vi "Actor Core.vi"(8 "error in":errorcluster, 11 "SCHEMA_01 in":refnum<class "SCHEMA_01.lvclass">) -> (0 "error out":errorcluster, 3 "Actor out":refnum<class "Actor.lvclass">)   [LabVIEW 2020, in "SCHEMA_01.lvlib" / "SCHEMA_01.lvclass"]
uses:
  SCHEMA_01.lvclass
  support/Actor Framework.lvlibp/1abvi3w/vi.lib/ActorFramework/Actor/Actor.lvclass
  D&C_SchemaBase/D&C_SchemaBase/D&C_SchemaBase.lvclass
panel:
  out "Source 1.T_0":dbl caption="Random.VAR 1" format="%#.1f"
  out "Source 1.T_6":dbl caption="Random.VAR 1" format="%#.1f"
  out "Source 1.T_5":dbl caption="Random.VAR 1" format="%#.1f"
  out "Source 1.T_4":dbl caption="Random.VAR 1" format="%#.1f"
  out "Source 1.T_3":dbl caption="Random.VAR 1" format="%#.1f"
  out "Source 1.T_2":dbl caption="Random.VAR 1" format="%#.1f"
  out "Source 1.T_1":dbl caption="Random.VAR 1" format="%#.1f"
  # "Source 1: les températures"
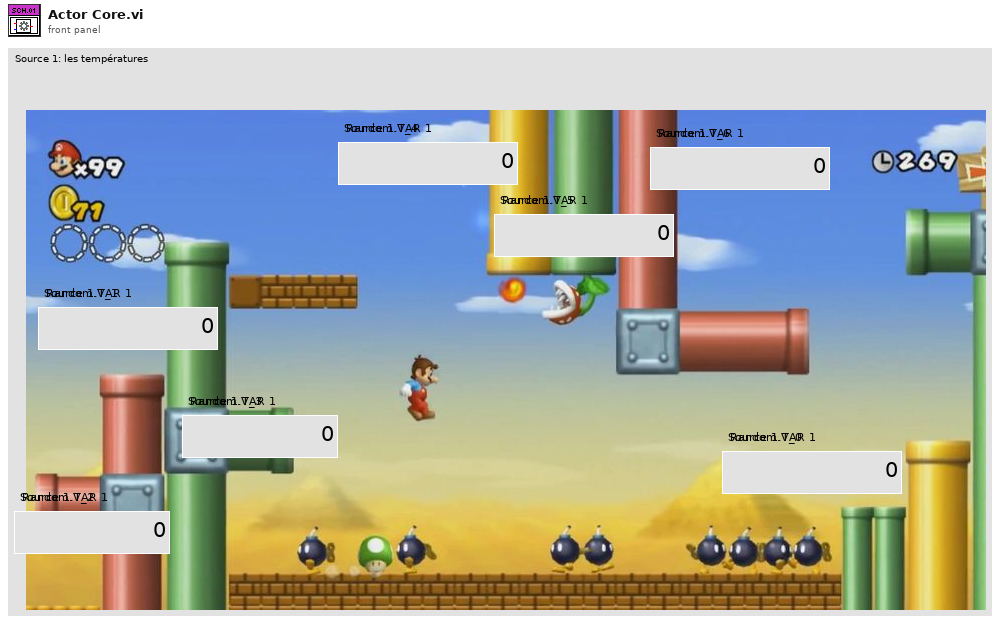
[diagram p1: front panel]
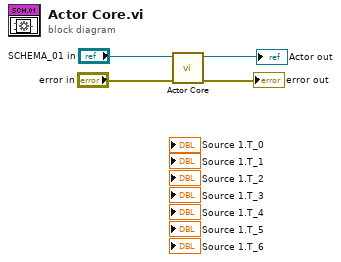
[diagram p0: block diagram]
diagram:
  n1 = call-parent "Actor Core.vi"("error in"="error in", "UI_Actor in"="SCHEMA_01 in") -> ("error out"=→"error out":errorcluster, "Actor out"=→"Actor out":refnum<class "Actor.lvclass">)  [unwired: 8 in]
